vi "GarageDoor_Create.vi"(8 "error in (no error)":errorcluster, 11 "reference in":refnum<class "GarageDoor.lvclass">) -> (0 "error out":errorcluster, 3 "reference out":refnum<class "GarageDoor.lvclass">)   [LabVIEW 2012, in "GarageDoor.lvclass"]
uses:
  GarageDoor.lvclass
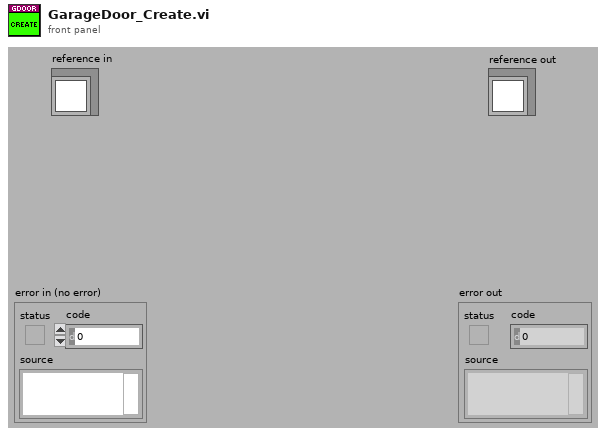
[diagram p1: front panel]
types:
  T1 = typedef "GarageDoor.lvclass/ObjectAttributes.ctl" = cluster{"None":bool}
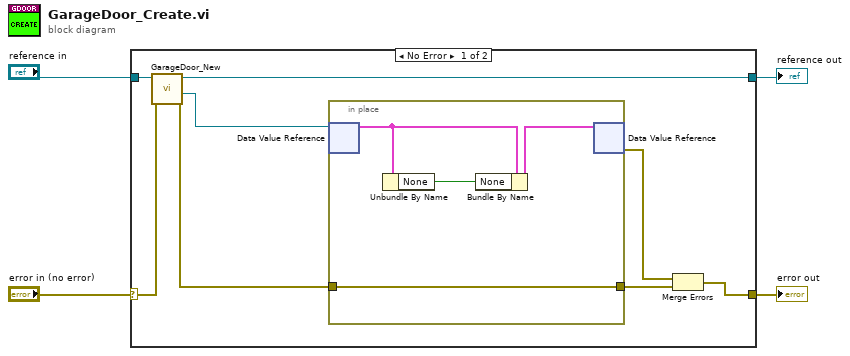
[diagram p0: block diagram]
diagram:
  n1 = case shown="No Error" "error in (no error)" {
    selector: "error in (no error)" -> [w11 w18]
    tunnel: [w8 w18] -> w3
    tunnel: "reference in" -> [w12 w17]
    tunnel: [w10 w17] -> w1
    frame No Error {
      n2 = call "GarageDoor_New.vi"("error in (no error)"=w11, "reference in"=w12) -> ("error out"=w6:errorcluster, "DVRRefOut"=w7:refnum<data-value>, "reference out"=w10:refnum<class "GarageDoor.lvclass">)  [unwired: 6 in, 1 out]
      n3 = in-place {
        in-place-border: w6 -> [w13]
        in-place-border: [w13] -> w5
        n4 = in-place-dvr #1(w7) -> (w15:T1)  [unwired: 1 out]
        n5 = Unbundle By Name(w15) -> ("None"=w14:bool)
        n6 = Bundle By Name(cluster=w15, "None"=w14) -> (w16:T1)
        n7 = in-place-dvr #1(w16) -> (w9:errorcluster)  [unwired: 1 out]
      }
      n8 = Merge Errors(w9, w5) -> (w8:errorcluster)
    }
    frame Error {
    }
  }
  "error out" <- w3
  "reference out" <- w1
